vi "Turret_Set.vi"   [LabVIEW 2019]
uses:
  Globals/Turret_Globals.vi
  Turret_States.ctl
  Robot Global Data.vi
  <vilib>/Rock Robotics/WPI/DriverStation/WPI_DriverStationRobotMode2.ctl
  Turret_Cluster.ctl
types:
  T1 = typedef "Turret_Cluster.ctl" = cluster{"Auto-Target?":bool, "Control_State":T2, "Turret_Spin_Speed":dbl, "Turret_Spin_Speed_Control?":bool, "Step":dbl, "Parameter_1":dbl, "Parameter_2":dbl, "Parameter_3":dbl, "Auto_Notifier":refnum<notifier>, "GoToZero?":bool}
  T2 = typedef "Turret_States.ctl" = enum16{"Manual_Percent_Voltage", "Manual_Speed_Control", "Auto-Target", "Command_TurnToPosition", "Command_Auto_Target", "GoToZero"}
  T3 = typedef "WPI_DriverStationRobotMode2.ctl" = enum16{"Autonomous Disabled", "Autonomous Enabled", "Teleop Disabled", "Teleop Enabled", "Disconnected", "Finish", "Test Disabled", "Test Enabled", "Emergency Stopped"}
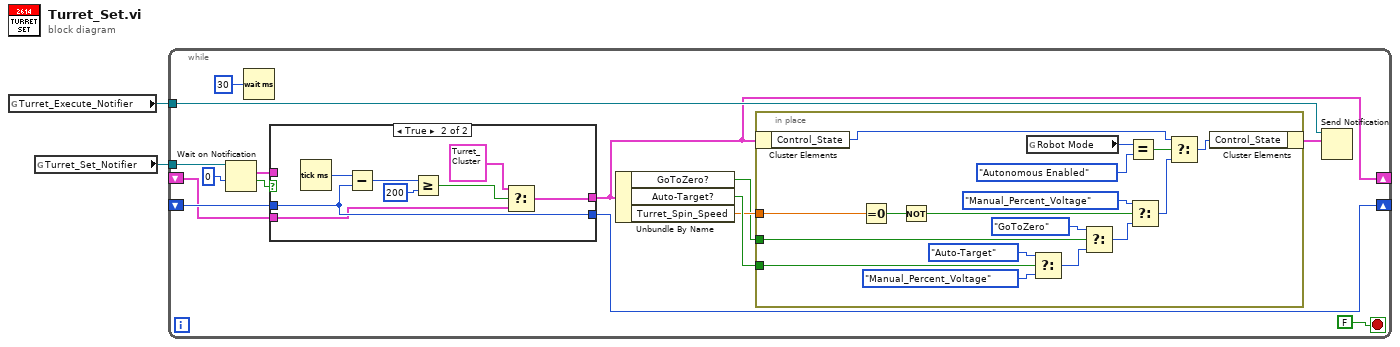
[diagram p0: block diagram]
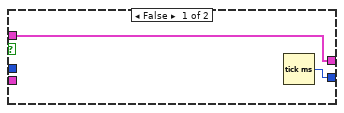
[diagram p2: hidden frame]
diagram:
  n1 = global read "Turret_Globals.vi" "Turret_Execute_Notifier"() -> (w1:refnum<notifier>)
  n2 = global read "Turret_Globals.vi" "Turret_Set_Notifier"() -> (w2:refnum<notifier>)
  n3 = while {
    tunnel: w2 -> [w15]
    tunnel: w1 -> [w13]
    shift-right: [w9] -> _
    shift-left: _ -> [w8]
    shift-right: [w5] -> _
    shift-left: _ -> [w4]
    stop <- FALSE stop-if-true
    n4 = Wait on Notification(notifier=w15, timeout in ms (-1)=0) -> (notification=w10:T1, timed out?=w7:bool)  [unwired: 2 in, 2 out]
    n5 = Wait (ms)(milliseconds to wait=u32 30) -> ()  [unwired: 1 out]
    n6 = case shown="True" w7 {
      tunnel: w10 -> [w19 _]
      tunnel: [w19 w22] -> w5
      tunnel: [w18 w26] -> w9
      tunnel: w8 -> [_ w26]
      tunnel: w4 -> [_ w20]
      frame False {
        n7 = Tick Count (ms)() -> (millisecond timer value=w18:u32)
      }
      frame True {
        n8 = Tick Count (ms)() -> (millisecond timer value=w27:u32)
        n9 = Subtract(x=w27, y=w26) -> (x-y=w25:u32)
        n10 = Greater Or Equal?(x=w25, y=u32 200) -> (x >= y?=w23:bool)
        n11 = Select(t=T1 {"Auto-Target?"=FALSE, "Control_State"=enum."Manual_Percent_Voltage", "Turret_Spin_Speed"=0.0, "Turret_Spin_Speed_Control?"=FALSE, "Step"=0.0, "Parameter_1"=0.0, "Parameter_2"=0.0, "Parameter_3"=0.0, "Auto_Notifier"=refnum, "GoToZero?"=FALSE} ("Turret_Cluster"), s=w23, f=w20) -> (s? t:f=w22:T1)
      }
    }
    n12 = Unbundle By Name(w5) -> ("GoToZero?"=w3:bool, "Auto-Target?"=w12:bool, "Turret_Spin_Speed"=w11:dbl)
    n13 = in-place {
      in-place-border: w12 -> [w42]
      in-place-border: w11 -> [w40]
      in-place-border: w3 -> [w30]
      n14 = in-place-cluster #1(w5) -> ("Control_State"=w33:T2)
      n15 = Equal To 0?(x=w40) -> (x = 0?=w39:bool)
      n16 = Not(x=w39) -> (.not. x?=w38:bool)
      n17 = global read "Robot Global Data.vi" "Robot Mode"() -> (w35:T3)
      n18 = Select(t=Turret_States."Auto-Target" ("Control_State"), s=w42, f=Turret_States."Manual_Percent_Voltage" ("Control_State")) -> (s? t:f=w28:T2)
      n19 = Select(t=Turret_States."GoToZero" ("Control_State"), s=w30, f=w28) -> (s? t:f=w31:T2)
      n20 = Equal?(x=w35, y=WPI_DriverStationRobotMode2."Autonomous Enabled") -> (x = y?=w36:bool)
      n21 = Select(t=Turret_States."Manual_Percent_Voltage", s=w38, f=w31) -> (s? t:f=w37:T2)
      n22 = Select(t=w33, s=w36, f=w37) -> (s? t:f=w32:T2)
      n23 = in-place-cluster #1("Control_State"=w32) -> (w14:T1)
    }
    n24 = Send Notification(notification=w14, notifier=w13) -> ()  [unwired: 1 in, 2 out]
  }
